vi "Update Verbose Explanation.vi"(9 "Overwrite":bool=TRUE, 10 "String":string, 11 "TestManagerMsg.Assertion in":refnum<class "TestManagerMsg.Assertion.lvclass">) -> (1 "Overwritten":bool, 3 "TestManagerMsg.Assertion out":refnum<class "TestManagerMsg.Assertion.lvclass">)   [LabVIEW 2013, in "Caraya.lvlib" / "TestManagerMsg.Assertion.lvclass"]
uses:
  TestManagerMsg.Assertion.lvclass
  TestManagerMsg.Assertion.lvclass/TestManagerMsg.Assertion.ctl
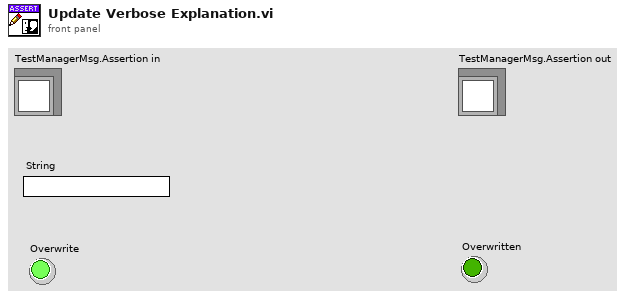
[diagram p1: front panel]
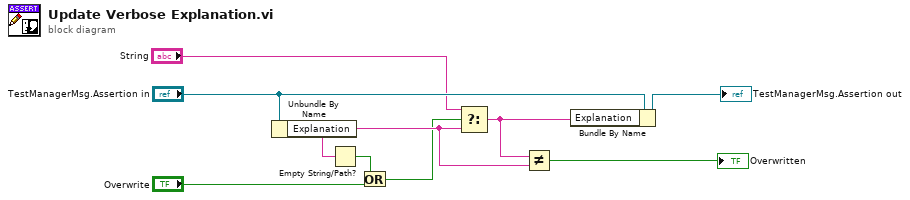
[diagram p0: block diagram]
diagram:
  n1 = Unbundle By Name("TestManagerMsg.Assertion in") -> ("Explanation"=w4:string)
  n2 = Empty String/Path?(string/path=w4) -> (empty?=w9:bool)
  n3 = Or(x=w9, y="Overwrite") -> (x .or. y?=w3:bool)
  n4 = Select(t="String", s=w3, f=w4) -> (s? t:f=w2:string)
  n5 = Not Equal?(x=w2, y=w4) -> (x != y?=→"Overwritten":bool)
  n6 = Bundle By Name(cluster="TestManagerMsg.Assertion in", "Explanation"=w2) -> (→"TestManagerMsg.Assertion out":refnum<class "TestManagerMsg.Assertion.lvclass">)
